vi "To Generic.vi"(8 "error in (no error)":errorcluster, 11 "Generic Data in":refnum<class "Generic Data.lvclass">) -> (0 "error out":errorcluster, 2 "Generic Data":refnum<class "Generic Data.lvclass">[](array[class]), 3 "Data Name":string[](array[string]))   [LabVIEW 2020, in "Data.lvlib" / "Generic Data.lvclass"]
doc: "Present private data as an array of named generic data elements."
uses:
  Generic Data.lvclass
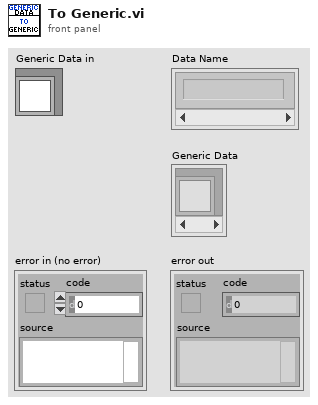
[diagram p1: front panel]
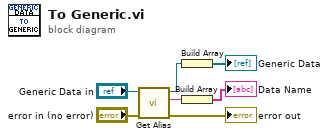
[diagram p0: block diagram]
diagram:
  n1 = call-dynamic "Get Alias.vi"("error in (no error)"="error in (no error)", "Data in"="Generic Data in") -> ("error out"=→"error out":errorcluster, "Alias"=w4:string, "Data out"=w6:refnum<class "Generic Data.lvclass">)  [unwired: 7 in]
  n2 = Build Array(w6) -> (→"Generic Data":refnum<class "Generic Data.lvclass">[])
  n3 = Build Array(w4) -> (→"Data Name":string[])
